vi "Get Documents.vi"(8 "error in (no error)":errorcluster, 11 "YAML Parser in":refnum<class "YAML Parser.lvclass">) -> (0 "error out":errorcluster, 1 "Not Found?":bool, 2 "Document String":string, 3 "YAML Parser out":refnum<class "YAML Parser.lvclass">)   [LabVIEW 2015, in "YAML Parser.lvclass"]
uses:
  YAML Parser.lvclass
  <vilib>/regexp/Match Regular Expression.xnode
panel:
  in  "Document Index":i32
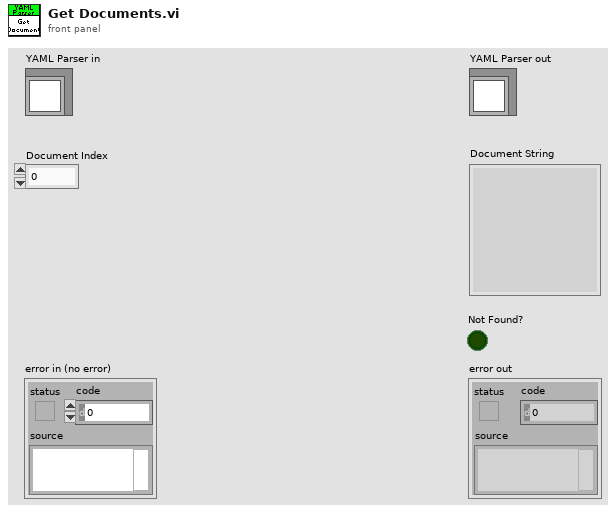
[diagram p1: front panel]
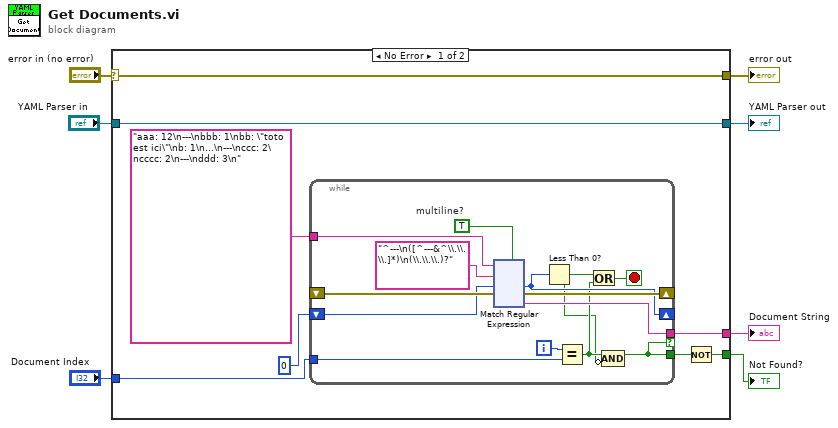
[diagram p0: block diagram]
diagram:
  n1 = case shown="No Error" "error in (no error)" {
    selector: "error in (no error)" -> [w14 w147]
    tunnel: [w14 w147] -> w6
    tunnel: [w15 w146] -> w4
    tunnel: "YAML Parser in" -> [w15 w146]
    tunnel: "Document Index" -> [w11 _]
    tunnel: [w10 _] -> w2
    tunnel: [w8 _] -> w1
    frame No Error {
      n2 = while {
        tunnel: "aaa: 12\n---\nbbb: 1\nbb: \"toto est ici\"\nb: 1\n...\n---\nccc: 2\ncccc: 2\n---\nddd: 3\n" -> [w26]
        shift-right: [w28] -> _
        shift-left: _ -> [w29]
        shift-right: [w23] -> _
        shift-left: 0 ("offset past match") -> [w24]
        tunnel: [w22] -> w10 if=w17
        tunnel: w11 -> [w20]
        tunnel: [w17] -> w9
        i -> [w21]
        stop <- w19 stop-if-true
        w25 = TRUE  # multiline?
        n3 = xnode "Match Regular Expression"("input string"=w26, "regular expression"="^---\n([^---&^\\.\\.\\.]*)\n(\\.\\.\\.)?", "offset (0)"=w24, "error in"=w29, "multiline? (F)"=w25) -> ("offset past match"=w23:i32, "error out"=w28:errorcluster, "submatch 1"=w22:string)  [unwired: 1 in, 3 out]
        n4 = Less Than 0?(x=w23) -> (x < 0?=w16:bool)
        n5 = Equal?(x=w21, y=w20) -> (x = y?=w18:bool)
        n6 = Or(x=w16, y=w18) -> (x .or. y?=w19:bool)
        n7 = Compound Arithmetic op=AND(w18, invert w16) -> (w17:bool)
      }
      n8 = Not(x=w9) -> (.not. x?=w8:bool)
    }
    frame Error {
    }
  }
  "error out" <- w6
  "YAML Parser out" <- w4
  "Document String" <- w2
  "Not Found?" <- w1
